vi "CheckReplyError.vi"(3 "error in":errorcluster, 4 "Response":T1, 5 "Error String":string) -> (0 "error out":errorcluster, 1 "APIs":string[](array[string]), 2 "Registered?":bool)   [LabVIEW 2016]
doc: "Checks for an error in the reply"
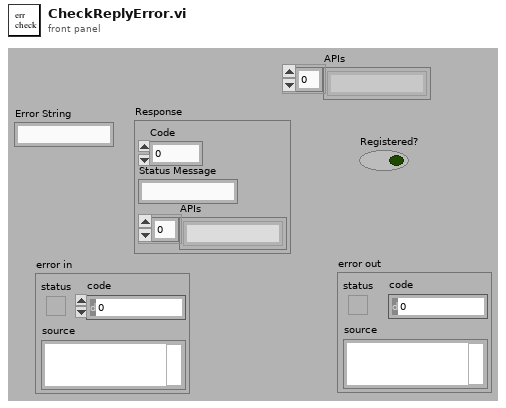
[diagram p1: front panel]
types:
  T1 = cluster{"Code":i32, "Status Message":string, "APIs":string[]}
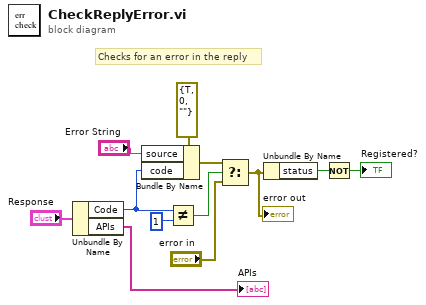
[diagram p0: block diagram]
diagram:
  # "Checks for an error in the reply"
  n1 = Unbundle By Name("Response") -> ("Code"=w4:i32, "APIs"=→"APIs":string[])
  n2 = Bundle By Name(cluster=errorcluster {"status"=TRUE, "code"=0, "source"=""} ("error out"), "source"="Error String", "code"=w4) -> (w5:errorcluster)
  n3 = Not Equal?(x=w4, y=1) -> (x != y?=w3:bool)
  n4 = Select(t=w5, s=w3, f="error in") -> (s? t:f=w10:errorcluster)
  "error out" <- w10
  n5 = Unbundle By Name(w10) -> ("status"=w11:bool)
  n6 = Not(x=w11) -> (.not. x?=→"Registered?":bool)
